vi "getGoodSetting.vi"(6 "addr/port":cluster{"address":string, "port":i32}={"address"="127.0.0.1", "port"=31415}, 8 "error in (no error)":errorcluster) -> (0 "error out":errorcluster, 3 "setting":dbl)   [LabVIEW 2015]
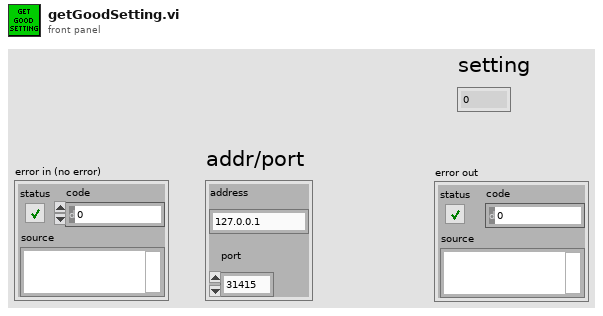
[diagram p1: front panel]
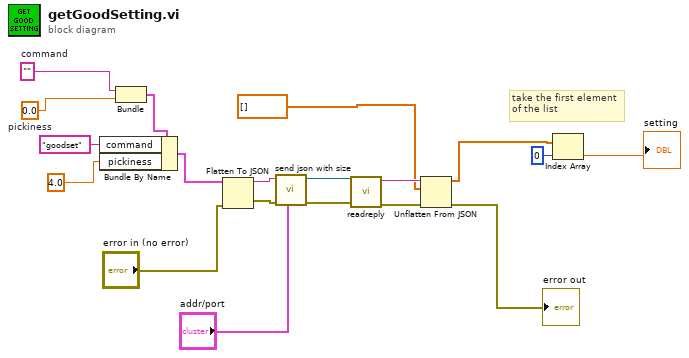
[diagram p0: block diagram]
diagram:
  w11 = 0.0  # pickiness
  w12 = ""  # command
  # "take the first element\nof the list"
  n1 = Bundle("command"=w12, "pickiness"=w11) -> (w10:cluster{"command":string, "pickiness":dbl})  [unwired: 1 in]
  n2 = Bundle By Name(cluster=w10, "command"="goodset", "pickiness"=4.0) -> (w5:cluster{"command":string, "pickiness":dbl})
  n3 = Flatten To JSON(anything=w5, error in (no error)="error in (no error)") -> (JSON string=w6:string, 11:w7:errorcluster)  [unwired: 1 in]
  n4 = call "send json with size.vi"("addr/port"="addr/port", "error in"=w7, "json string"=w6) -> ("error out"=w2:errorcluster, "connection ID out"=w1:refnum<k5>)  [unwired: 6 in, 1 out]
  n5 = call "readreply.vi"("error in (no error)"=w2, "connection ID"=w1) -> ("error out"=w19:errorcluster, "data out"=w17:string)  [unwired: 8 in]
  n6 = Unflatten From JSON(JSON string=w17, type and defaults=dbl[] [] ("Array"), error in (no error)=w19) -> (value=w13:dbl[], error out=→"error out":errorcluster)  [unwired: 4 in]
  n7 = Index Array(array=w13, index=0) -> (element=→"setting":dbl)
